vi "E517_Initialisation.vi"(11 "error out":errorcluster) -> (4 "Position":dbl[](array[numeric]) format="%.6f", 6 "Identification":string, 8 "Conn. Axes":string[](array[string]), 15 "error out 2":errorcluster)   [LabVIEW 2013]
uses:
  Utilities/controls/ctlSeqFNs_PI_SysNr.ctl
  Variables/GlobalSetGetPositionParameters.vi
  Variables/GlobalSetConfigurationPhysikalInstruments.vi
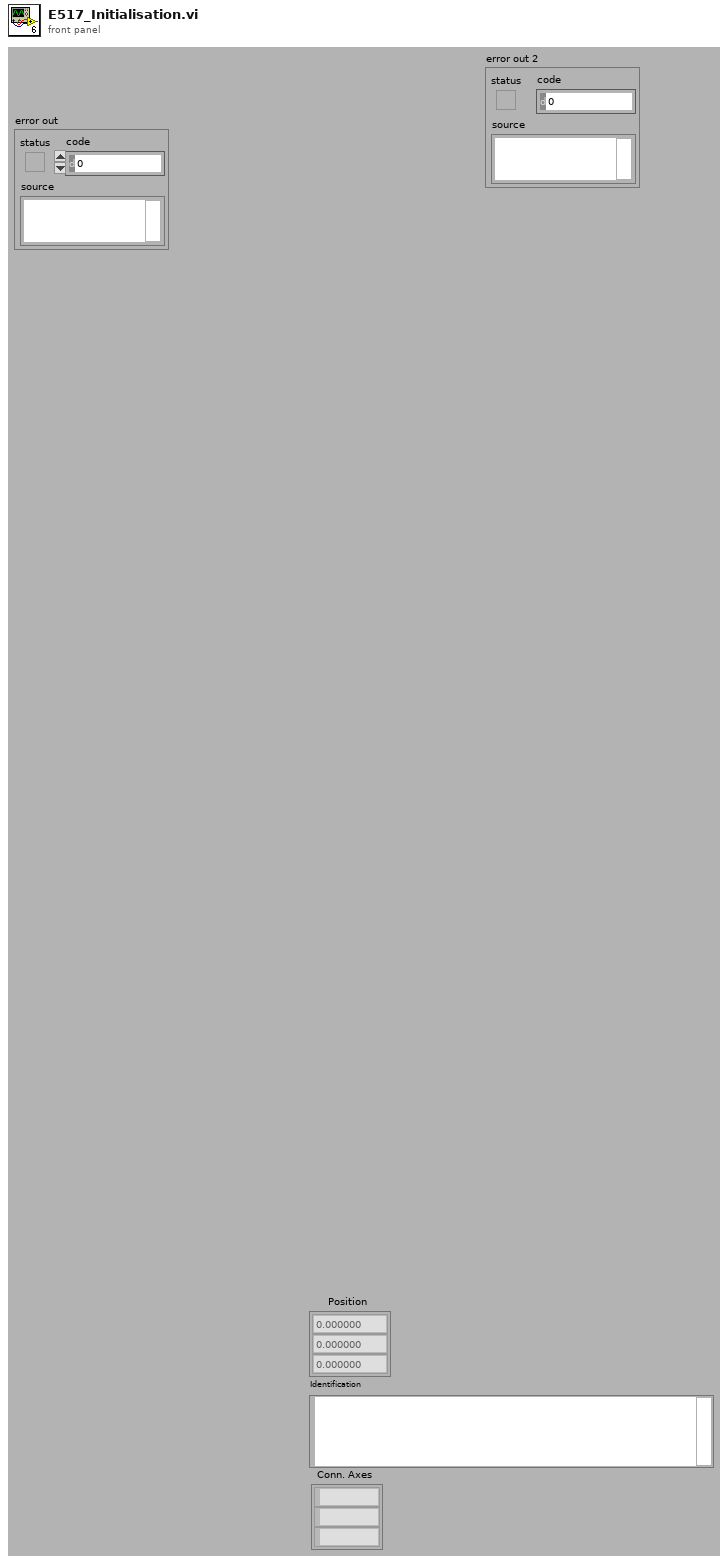
[diagram p1: front panel]
types:
  T1 = typedef "ctlSeqFNs_PI_SysNr.ctl" = enum16{"Zero", "E517", "E710"}
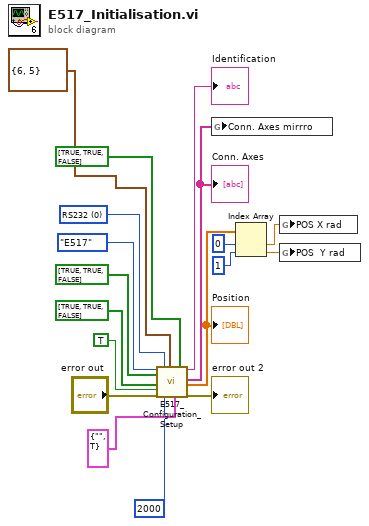
[diagram p0: block diagram]
diagram:
  w14 = u16 0 items=["RS232", "GPIB", "TCP/IP", "USB"] ("Interface")
  n1 = call "E517_Configuration_Setup.vi"("System no."=ctlSeqFNs_PI_SysNr."E517" ("STATE"), "Set channel online?"=bool[] [TRUE, TRUE, FALSE], "Switch servo on?"=bool[] [TRUE, TRUE, FALSE], "Stop wave generator\noutput (if any)"=TRUE ("Stop wave generator\noutput (if any)"), "error in"="error out", "Interface"=w14, "Timeout"=u32 2000, "RS232 settings"=cluster{"Portnumber":i32, "Baudrate":u16} {"Portnumber"=6, "Baudrate"=5}, "USB settings"=cluster{"S/N":string, "USB Search?":bool} {"S/N"="", "USB Search?"=TRUE}, "Axes to move to middle"=bool[] [TRUE, TRUE, FALSE]) -> ("Identification"=→"Identification":string, "Conn. Axes"=w10:string[], "Position"=w11:dbl[], "error out"=→"error out 2":errorcluster)  [unwired: 4 in, 2 out]
  "Position" <- w11
  "Conn. Axes" <- w10
  n2 = global write "GlobalSetConfigurationPhysikalInstruments.vi" "Conn. Axes mirrro"(w10) -> ()
  n3 = Index Array(array=w11, index #1=0 ("index"), index #2=1 ("index")) -> (element #1=w4:dbl, element #2=w5:dbl)
  n4 = global write "GlobalSetGetPositionParameters.vi" "POS X rad"(w4) -> ()
  n5 = global write "GlobalSetGetPositionParameters.vi" "POS  Y rad"(w5) -> ()
